vi "Configure Trigger.vi"(6 "Manual Trigger Delay (5.0 s)":dbl=5.0 format="%.2f", 8 "error in (no error)":errorcluster, 9 "Default Trigger Delay (True)":bool=TRUE, 10 "Trigger Source (0: Internal)":u16(ring) items=["Internal", "External"], 11 "VISA resource name":refnum<visa-resource-name>) -> (0 "error out":errorcluster, 3 "VISA resource name out":refnum<visa-resource-name>)   [LabVIEW 2012, in "Fluke 8508.lvlib"]
doc: "This VI configures the trigger settings on the instrument."
uses:
  Fluke 8508.lvlib
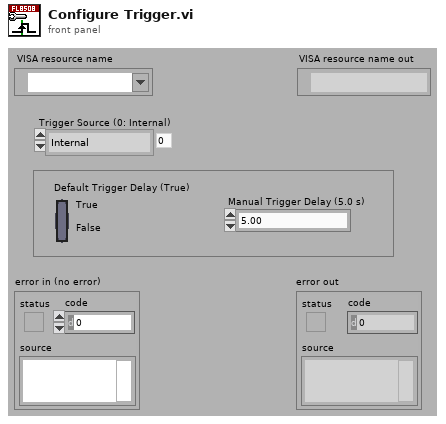
[diagram p1: front panel]
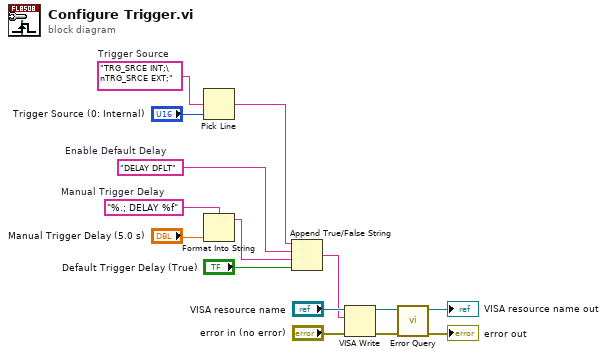
[diagram p0: block diagram]
diagram:
  w8 = "DELAY DFLT"  # Enable Default Delay
  w9 = "%.; DELAY %f"  # Manual Trigger Delay
  w14 = "TRG_SRCE INT;\nTRG_SRCE EXT;"  # Trigger Source
  n1 = Pick Line(multi-line string=w14, line index="Trigger Source (0: Internal)") -> (output string=w6:string)  [unwired: 1 in]
  n2 = Format Into String(format string=w9, "Manual Trigger Delay (5.0 s)") -> (resulting string=w7:string)  [unwired: 2 in, 1 out]
  n3 = Append True/False String(1:"Default Trigger Delay (True)", 2:w7, 3:w8, 4:w6) -> (0:w5:string)
  n4 = VISA Write(VISA resource name="VISA resource name", write buffer=w5, error in (no error)="error in (no error)") -> (VISA resource name out=w3:refnum<visa-resource-name>, error out=w4:errorcluster)  [unwired: 1 out]
  n5 = call "Error Query.vi"("error in (no error)"=w4, "VISA resource name"=w3) -> ("error out"=→"error out":errorcluster, "VISA resource name out"=→"VISA resource name out":refnum<visa-resource-name>)  [unwired: 6 in, 2 out]
